vi "FTW-ActorExtended-Publisher-Add.vi"(0 "FTW-ActorExtended In":refnum<class "FTW-ActorExtended.lvclass">, 5 "Publisher Name":string, 7 "Publisher URI":string, 11 "error in":errorcluster, 12 "Send Buffer Depth (1)":i32=1, 13 "Send Timeout (-1)":i32=-1) -> (4 "FTW-ActorExtended Out":refnum<class "FTW-ActorExtended.lvclass">, 15 "error out":errorcluster)   [LabVIEW 2015, in "FTW-ActorExtended.lvclass"]
uses:
  FTW-ActorExtended.lvclass
  FTW-ActorExtended.lvclass/FTW-ActorExtended.ctl
  Publisher/FTW-Publisher.lvclass
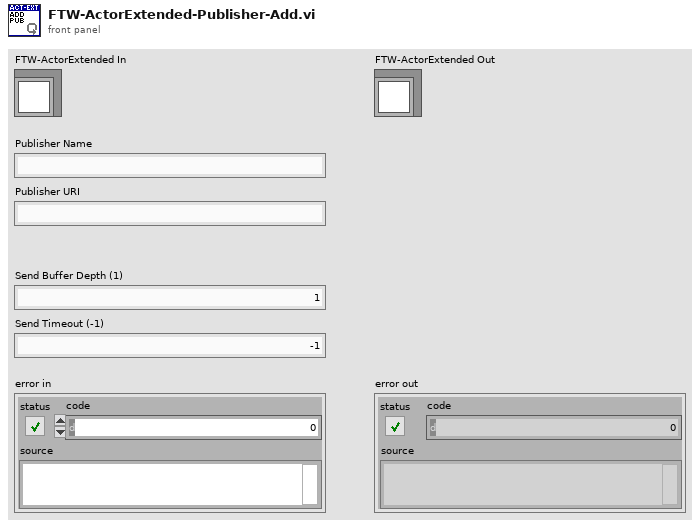
[diagram p1: front panel]
types:
  T1 = cluster{"Name":string, "URI":string, "Publisher":refnum<class "FTW-Publisher.lvclass">}[]
  T2 = cluster{"Publisher Name":string, "Actual Address":string, "FTW-Publisher Out":refnum<class "FTW-Publisher.lvclass">}
  T3 = cluster{"Publisher Name":string, "Actual Address":string, "FTW-Publisher Out":refnum<class "FTW-Publisher.lvclass">}[]
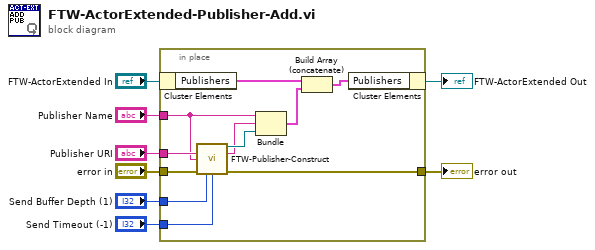
[diagram p0: block diagram]
diagram:
  n1 = in-place {
    in-place-border: "Publisher URI" -> [w19]
    in-place-border: "Publisher Name" -> [w15]
    in-place-border: "Send Buffer Depth (1)" -> [w12]
    in-place-border: "Send Timeout (-1)" -> [w11]
    in-place-border: [w10] -> w2
    in-place-border: "error in" -> [w9]
    n2 = in-place-cluster #1("FTW-ActorExtended In") -> ("Publishers"=w16:T1)
    n3 = call "FTW-Publisher-Construct.vi"("Address"=w19, "Identity"=w15, "error in"=w9, "Send Buffer Depth (1)"=w12, "Send Timeout (-1)"=w11) -> ("FTW-Publisher Out"=w14:refnum<class "FTW-Publisher.lvclass">, "Actual Address"=w13:string, "error out"=w10:errorcluster)  [unwired: 8 in]
    n4 = Bundle("Publisher Name"=w15, "Actual Address"=w13, "FTW-Publisher Out"=w14) -> (w18:T2)  [unwired: 1 in]
    n5 = Build Array (concatenate)(w16, w18) -> (w17:T3)
    n6 = in-place-cluster #1("Publishers"=w17) -> (→"FTW-ActorExtended Out":refnum<class "FTW-ActorExtended.lvclass">)
  }
  "error out" <- w2
